vi "Periodic Tasks.vi"(8 "error in":errorcluster) -> ()   [LabVIEW 2019]
doc: "This VI runs in parallel to other robot code. It can contain as many user-defined periodic loops as you need. These can carry out PID or other sorts of timed response."
uses:
  <vilib>/Rock Robotics/Network Tables/NT Write String Array.vi
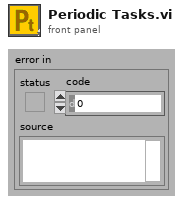
[diagram p1: front panel]
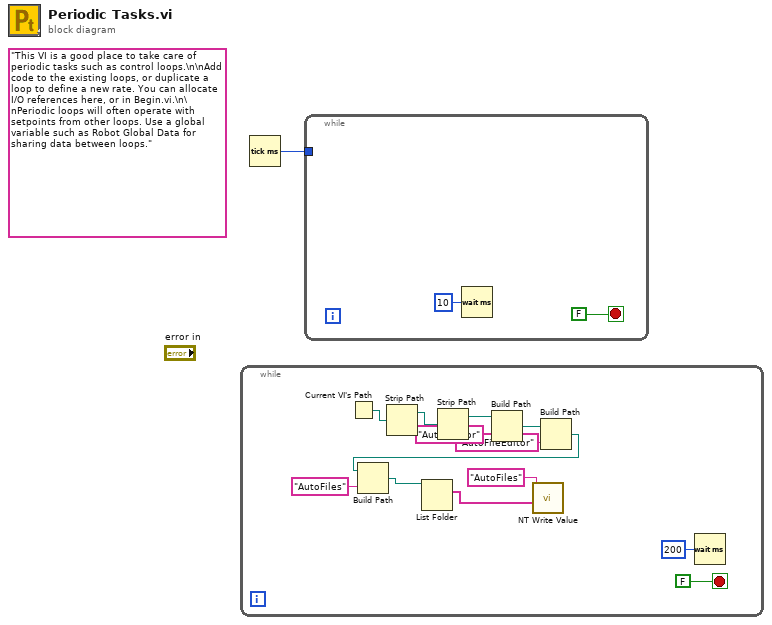
[diagram p0: block diagram]
diagram:
  (unwired) "This VI is a good place to take care of periodic tasks such as control loops.\n\nAdd code to the existing loops, or duplicate a loop to define a new rate. You can allocate I/O references here, or in Begin.vi.\n\nPeriodic loops will often operate with setpoints from other loops. Use a global variable such as Robot Global Data for sharing data between loops."
  n1 = while {
    stop <- FALSE stop-if-true
    n2 = Current VI's Path() -> (path=w12:path)
    n3 = Strip Path(path=w12) -> (stripped path=w11:path)  [unwired: 1 out]
    n4 = Strip Path(path=w11) -> (stripped path=w10:path)  [unwired: 1 out]
    n5 = Build Path(base path=w10, name or relative path="Auto Editor") -> (appended path=w9:path)
    n6 = Build Path(base path=w9, name or relative path="AutoFileEditor") -> (appended path=w8:path)
    n7 = Build Path(base path=w8, name or relative path="AutoFiles") -> (appended path=w4:path)
    n8 = List Folder(path=w4) -> (filenames=w3:string[])  [unwired: 3 in, 3 out]
    n9 = call-poly <vilib>:"NT Write Value.vi"("String Array"=w3, "Name"="AutoFiles") -> ()  [unwired: 9 in, 1 out]
    n10 = Wait (ms)(milliseconds to wait=u32 200) -> ()  [unwired: 1 out]
  }
  n11 = Tick Count (ms)() -> (millisecond timer value=w1:u32)
  n12 = while {
    tunnel: w1 -> [_]
    stop <- FALSE stop-if-true
    n13 = Wait (ms)(milliseconds to wait=u32 10) -> ()  [unwired: 1 out]
  }
